vi "CAL_Power_R.vi"(0 "Stride?":bool, 2 "Positive Power":sgl[](array[numeric]), 3 "출력 클러스터 2":T1, 4 "Period_R":sgl) -> (7 "R_power_OK":bool, 9 "CAN":enum16{"stand", "init", "read"}(ring), 10 "출력 클러스터 3":T1)   [LabVIEW 2019]
uses:
  fa2a1903-695d-47df-94d3-5e85488a5f8b.vi
panel:
  in  "R_power_OK 2":bool
  in  "Negative Powe":sgl[](array[numeric])
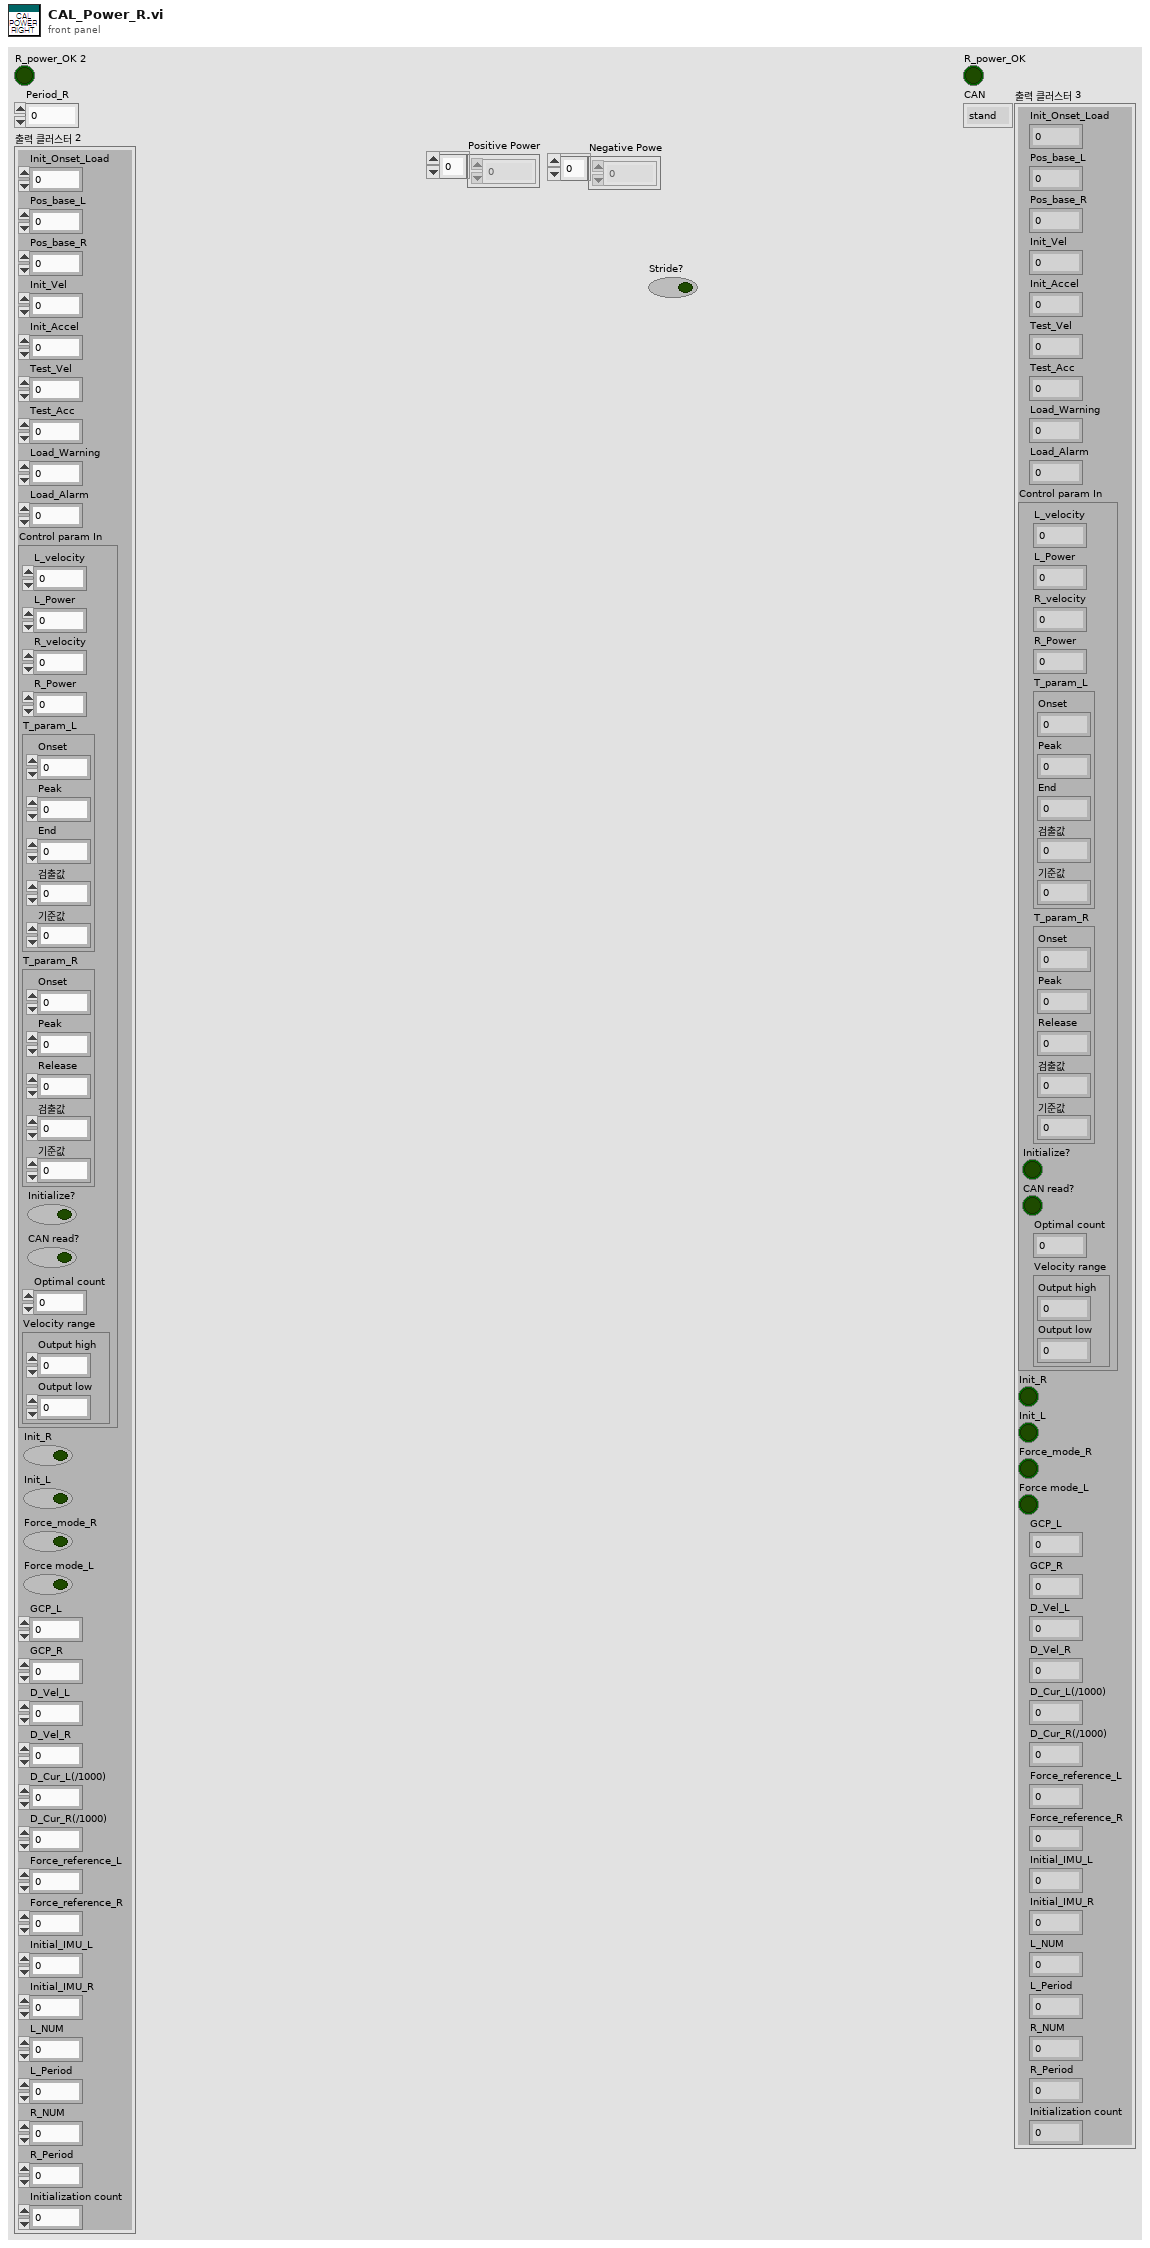
[diagram p1: front panel]
types:
  T1 = cluster{"Init_Onset_Load":sgl, "Pos_base_L":sgl, "Pos_base_R":sgl, "Init_Vel":i32, "Init_Accel":u32, "Test_Vel":i32, "Test_Acc":u32, "Load_Warning":sgl, "Load_Alarm":sgl, "Control param In":cluster{"L_velocity":u32, "L_Power":sgl, "R_velocity":u32, "R_Power":sgl, "T_param_L":cluster{"Onset":sgl, "Peak":sgl, "End":sgl, "검출값":sgl, "기준값":sgl}, "T_param_R":cluster{"Onset":sgl, "Peak":sgl, "Release":sgl, "검출값":sgl, "기준값":sgl}, "Initialize?":bool, "CAN read?":bool, "Optimal count":i32, "Velocity range":cluster{"Output high":dbl, "Output low":dbl}}, "Init_R":bool, "Init_L":bool, "Force_mode_R":bool, "Force mode_L":bool, "GCP_L":sgl, "GCP_R":sgl, "D_Vel_L":sgl, "D_Vel_R":sgl, "D_Cur_L(/1000)":sgl, "D_Cur_R(/1000)":sgl, "Force_reference_L":sgl, "Force_reference_R":sgl, "Initial_IMU_L":sgl, "Initial_IMU_R":sgl, "L_NUM":u32, "L_Period":i16, "R_NUM":u32, "R_Period":i16, "Initialization count":i32}
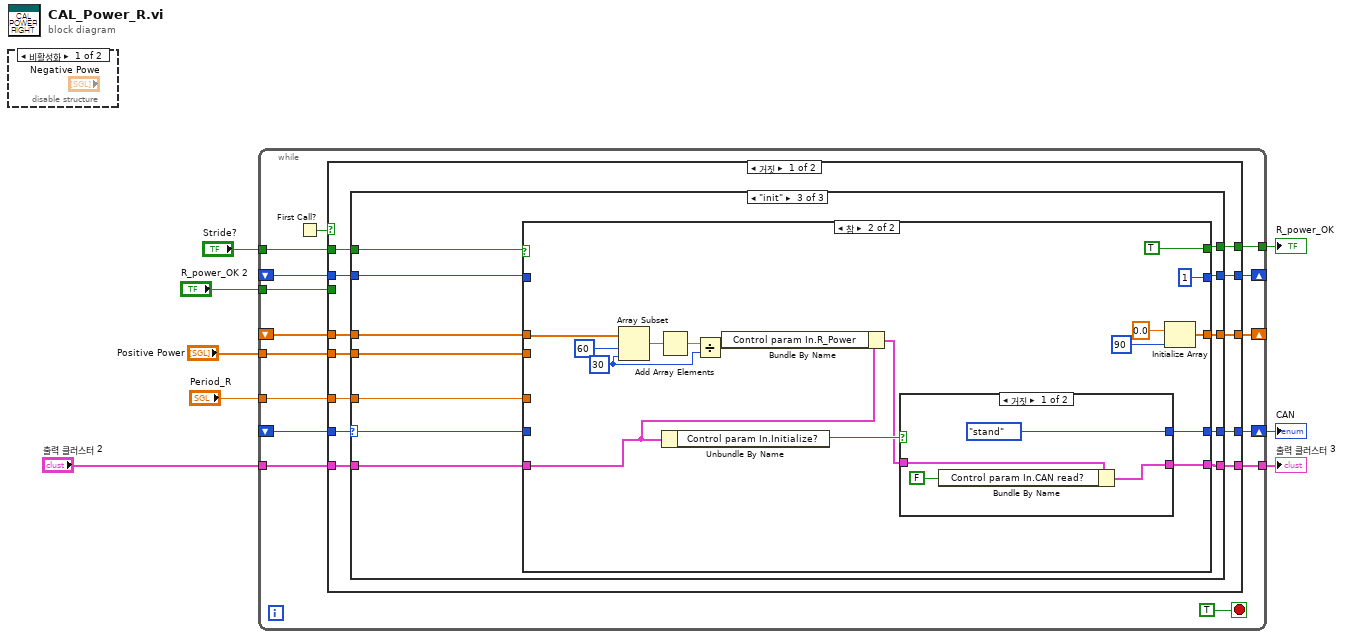
[diagram p0: block diagram]
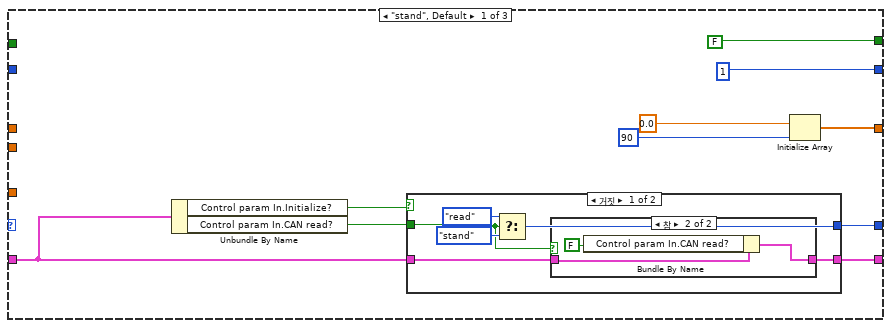
[diagram p3: hidden frame]
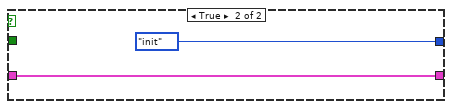
[diagram p5: hidden frame]
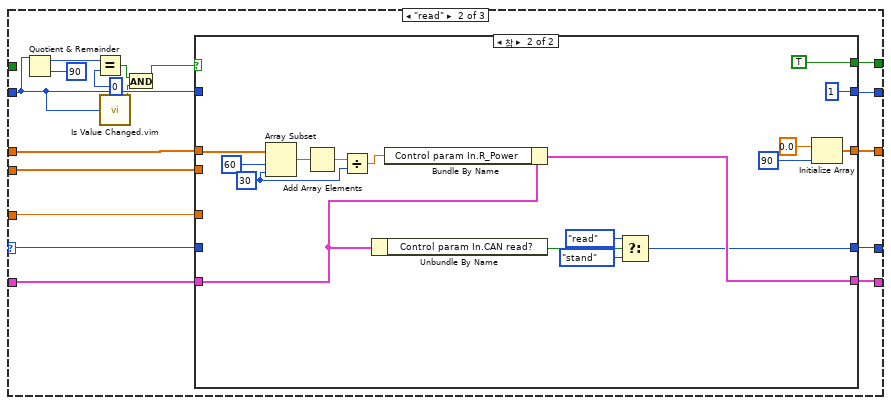
[diagram p6: hidden frame]
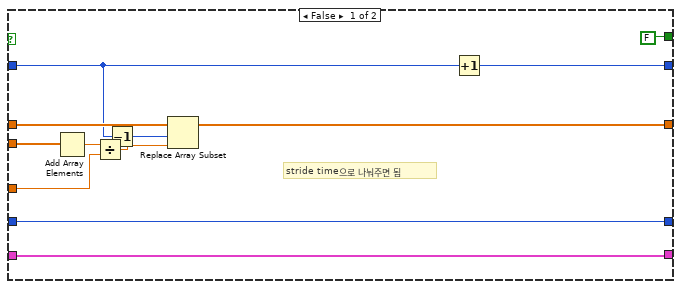
[diagram p7: hidden frame]
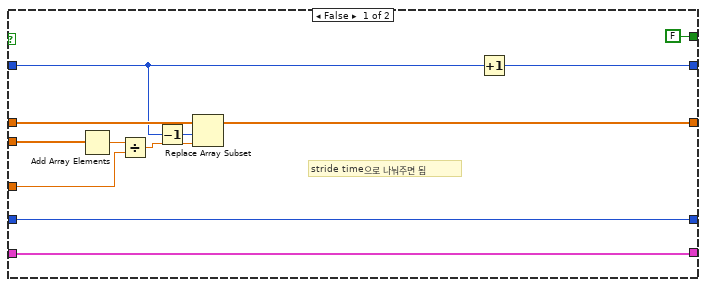
[diagram p8: hidden frame]
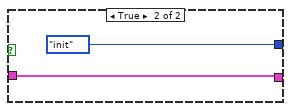
[diagram p9: hidden frame]
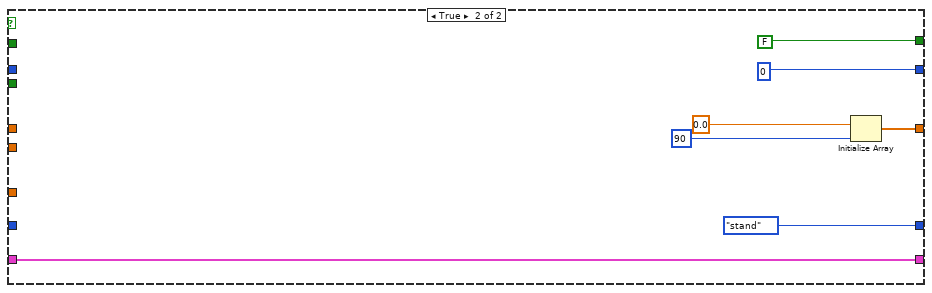
[diagram p10: hidden frame]
diagram:
  n1 = disable-structure shown="비활성화" {
    frame Disabled {
    }
    frame Enabled {
    }
  }
  n2 = while {
    tunnel: "Positive Power" -> [w17]
    shift-right: [w21] -> _
    shift-left: _ -> [w20]
    shift-right: [w19] -> _
    shift-left: _ -> [w18]
    tunnel: "출력 클러스터 2" -> [w16]
    tunnel: [w15] -> w1
    tunnel: [w14] -> w7
    tunnel: "R_power_OK 2" -> [w13]
    tunnel: "Stride?" -> [w12]
    tunnel: "Period_R" -> [w11]
    shift-right: [w10] -> w3
    shift-left: _ -> [w9]
    stop <- TRUE stop-if-true
    n3 = First Call?() -> (First Call?: T/F=w22:bool)
    n4 = case shown="거짓" w22 {
      tunnel: [w35 0] -> w21
      tunnel: w20 -> [w34 _]
      tunnel: [w31 w153] -> w19
      tunnel: w18 -> [w33 _]
      tunnel: w17 -> [w32 _]
      tunnel: w16 -> [w26 w152]
      tunnel: [w30 w152] -> w15
      tunnel: [w29 FALSE] -> w14
      tunnel: w13 -> [_ _]
      tunnel: w12 -> [w28 _]
      tunnel: w11 -> [w27 _]
      tunnel: [w25 enum16{"stand", "init", "read"}."stand" ("CAN")] -> w10
      tunnel: w9 -> [w24 _]
      frame False {
        n5 = case shown="\"init\"" w24 {
          selector: w24 -> [_ w71 w105]
          tunnel: [1 w69 w115] -> w35
          tunnel: w34 -> [_ w61 w114]
          tunnel: w33 -> [_ w74 w113]
          tunnel: w32 -> [_ w73 w112]
          tunnel: [w41 w70 w111] -> w31
          tunnel: [w36 w66 w110] -> w30
          tunnel: [FALSE w68 w109] -> w29
          tunnel: w28 -> [_ _ w108]
          tunnel: w27 -> [_ w72 w107]
          tunnel: w26 -> [w37 w62 w106]
          tunnel: [w40 w67 w104] -> w25
          frame "stand", Default {
            n6 = Unbundle By Name(w37) -> ("Control param In.Initialize?"=w39:bool, "Control param In.CAN read?"=w38:bool)
            n7 = case shown="거짓" w39 {
              tunnel: [w49 enum16{"stand", "init", "read"}."init" ("CAN")] -> w40
              tunnel: w38 -> [w48 _]
              tunnel: w37 -> [w47 w56]
              tunnel: [w46 w56] -> w36
              frame False {
                n8 = Select(t=enum16{"stand", "init", "read"}."read" ("CAN"), s=w48, f=enum16{"stand", "init", "read"}."stand" ("CAN")) -> (s? t:f=w49:enum16{"stand", "init", "read"})
                n9 = case shown="참" w48 {
                  tunnel: w47 -> [w52 w55]
                  tunnel: [w52 w54] -> w46
                  frame False {
                  }
                  frame True {
                    n10 = Bundle By Name(cluster=w55, "Control param In.CAN read?"=FALSE ("CAN read?")) -> (w54:T1)
                  }
                }
              }
              frame True {
              }
            }
            n11 = Initialize Array(sgl 0.0 ("원소"), 90 ("차원 크기")) -> (w41:sgl[])
          }
          frame "read" {
            n12 = Quotient & Remainder(x=w61, y=u32 90) -> (x-y*floor(x/y)=w64:u32)  [unwired: 1 out]
            n13 = Equal?(x=w64, y=u32 0) -> (x = y?=w60:bool)
            n14 = call "Is Value Changed.vim"("value"=w61) -> ("changed or first call?"=w59:bool)
            n15 = And(x=w60, y=w59) -> (x .and. y?=w58:bool)
            n16 = case shown="참" w58 {
              tunnel: [w86 1 ("y")] -> w69
              tunnel: w61 -> [w76 _]
              tunnel: w74 -> [w85 w97]
              tunnel: w73 -> [w81 _]
              tunnel: [w84 w100] -> w70
              tunnel: [w83 w99] -> w66
              tunnel: w62 -> [w83 w89]
              tunnel: [FALSE TRUE] -> w68
              tunnel: w72 -> [w79 _]
              tunnel: w71 -> [w77 _]
              tunnel: [w77 w92] -> w67
              frame False {
                # "stride time으로 나눠주면 됨"
                n17 = Add Array Elements(numeric array=w81) -> (sum=w80:sgl)
                n18 = Divide(x=w80, y=w79) -> (x/y=w78:sgl)
                n19 = Decrement(x=w76) -> (x-1=w75:i32)
                n20 = Replace Array Subset(array=w85, new element=w78, index=w75) -> (w84:sgl[])
                n21 = Increment(x=w76) -> (x+1=w86:i32)
              }
              frame True {
                w93 = 30 ("길이")
                n22 = Array Subset(array=w97, index=60 ("인덱스"), length=w93) -> (w95:sgl[])
                n23 = Add Array Elements(numeric array=w95) -> (sum=w94:sgl)
                n24 = Divide(x=w94, y=w93) -> (x/y=w87:sgl)
                n25 = Unbundle By Name(w89) -> ("Control param In.CAN read?"=w88:bool)
                n26 = Bundle By Name(cluster=w89, "Control param In.R_Power"=w87) -> (w99:T1)
                n27 = Select(t=enum16{"stand", "init", "read"}."read" ("CAN"), s=w88, f=enum16{"stand", "init", "read"}."stand" ("CAN")) -> (s? t:f=w92:enum16{"stand", "init", "read"})
                n28 = Initialize Array(sgl 0.0 ("원소"), 90 ("차원 크기")) -> (w100:sgl[])
              }
            }
          }
          frame "init" {
            n29 = case shown="참" w108 {
              tunnel: [w127 1 ("y")] -> w115
              tunnel: w114 -> [w117 _]
              tunnel: w113 -> [w126 w138]
              tunnel: w112 -> [w122 _]
              tunnel: [w125 w140] -> w111
              tunnel: [w124 w129] -> w110
              tunnel: w106 -> [w124 w132]
              tunnel: [FALSE TRUE] -> w109
              tunnel: w107 -> [w120 _]
              tunnel: w105 -> [w118 _]
              tunnel: [w118 w133] -> w104
              frame False {
                # "stride time으로 나눠주면 됨"
                n30 = Add Array Elements(numeric array=w122) -> (sum=w121:sgl)
                n31 = Divide(x=w121, y=w120) -> (x/y=w119:sgl)
                n32 = Decrement(x=w117) -> (x-1=w116:i32)
                n33 = Replace Array Subset(array=w126, new element=w119, index=w116) -> (w125:sgl[])
                n34 = Increment(x=w117) -> (x+1=w127:i32)
              }
              frame True {
                w134 = 30 ("길이")
                n35 = Array Subset(array=w138, index=60 ("인덱스"), length=w134) -> (w136:sgl[])
                n36 = Add Array Elements(numeric array=w136) -> (sum=w135:sgl)
                n37 = Unbundle By Name(w132) -> ("Control param In.Initialize?"=w131:bool)
                n38 = Divide(x=w135, y=w134) -> (x/y=w128:sgl)
                n39 = Bundle By Name(cluster=w132, "Control param In.R_Power"=w128) -> (w130:T1)
                n40 = case shown="거짓" w131 {
                  tunnel: [enum16{"stand", "init", "read"}."stand" ("CAN") enum16{"stand", "init", "read"}."init" ("CAN")] -> w133
                  tunnel: w130 -> [w146 w148]
                  tunnel: [w145 w148] -> w129
                  frame False {
                    n41 = Bundle By Name(cluster=w146, "Control param In.CAN read?"=FALSE ("CAN read?")) -> (w145:T1)
                  }
                  frame True {
                  }
                }
                n42 = Initialize Array(sgl 0.0 ("원소"), 90 ("차원 크기")) -> (w140:sgl[])
              }
            }
          }
        }
      }
      frame True {
        n43 = Initialize Array(sgl 0.0 ("원소"), 90 ("차원 크기")) -> (w153:sgl[])
      }
    }
  }
  "R_power_OK" <- w7
  "CAN" <- w3
  "출력 클러스터 3" <- w1
